vi "AB_Convert_To_Relative_Path.vi"(11 "absolute path":path) -> (3 "relative path":path)   [LabVIEW 2020]
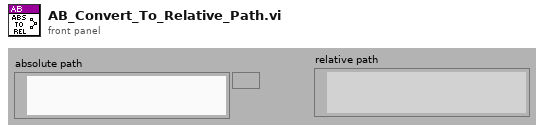
[diagram p1: front panel]
types:
  T1 = enum32{"invalid OS target", "Mac OS", "Windows 3.1", "Windows 95/NT", "Solaris 1", "Solaris 2", "HP-UX", "PowerMAX", "Linux", "Irix", "Rhapsody", "BeOS", "AIX", "OSF1", "VxWorks", "PharLap", "Carbon", "RTX", "Windows x64", "Linux x64", "Mac OS X x64"}
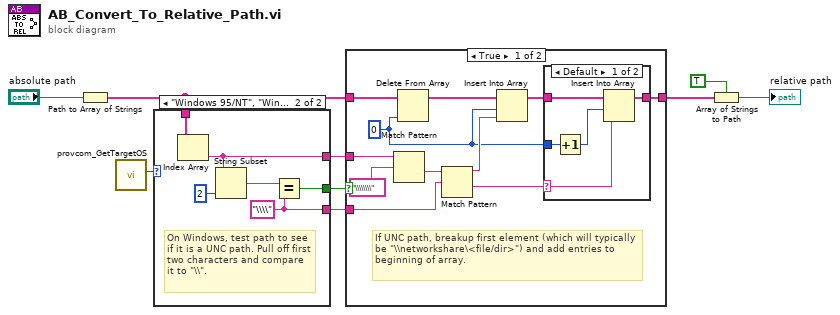
[diagram p0: block diagram]
diagram:
  n1 = Path to Array of Strings(0:"absolute path") -> (2:w7:string[])  [unwired: 1 out]
  n2 = call <resource>:"provcom_GetTargetOS.vi"() -> ("App.TargetOS"=w1:T1)  [unwired: 11 out]
  n3 = case shown="\"Windows 95/NT\", \"Windows x64\"" w1 {
    tunnel: [_ w13] -> w8
    tunnel: w7 -> [_ w12]
    tunnel: [_ w11] -> w5
    tunnel: [_ w10] -> w2
    frame Default {
    }
    frame "Windows 95/NT", "Windows x64" {
      w10 = "\\\\" ("regular expression")
      # "On Windows, test path to see if it is a UNC path. Pull off first two characters and compare it to \"\\\\\"."
      n4 = Index Array(array=w12) -> (element=w11:string)  [unwired: 1 in]
      n5 = String Subset(string=w11, length (rest)=2 ("length (rest)")) -> (substring=w14:string)  [unwired: 1 in]
      n6 = Equal?(x=w14, y=w10) -> (x = y?=w13:bool)
    }
  }
  n7 = case shown="True" w8 {
    tunnel: w7 -> [w26 w33]
    tunnel: [w17 w33] -> w6
    tunnel: w5 -> [w24 _]
    tunnel: w2 -> [w20 _]
    frame True {
      w16 = 0 ("index")
      # "If UNC path, breakup first element (which will typically be \"\\\\networkshare\\<file/dir>\") and add entries to beginning of array."
      n8 = Match Pattern(string=w24, regular expression="\\\\\\\\") -> (after substring=w23:string)  [unwired: 1 in, 3 out]
      n9 = Delete From Array(array=w26, index=w16) -> (array with subset deleted=w25:string[])  [unwired: 1 in, 1 out]
      n10 = Match Pattern(string=w23, regular expression=w20) -> (before substring=w22:string, after substring=w18:string)  [unwired: 1 in, 2 out]
      n11 = Insert Into Array(array=w25, index=w16, new element=w22) -> (w19:string[])
      n12 = case shown="Default" w18 {
        selector: w18 -> [w29 _]
        tunnel: w19 -> [w31 w32]
        tunnel: [w30 w32] -> w17
        tunnel: w16 -> [w28 _]
        frame Default {
          n13 = Increment(x=w28) -> (x+1=w27:i32)
          n14 = Insert Into Array(array=w31, index=w27, new element=w29) -> (w30:string[])
        }
        frame "" {
        }
      }
    }
    frame False {
    }
  }
  n15 = Array of Strings to Path(0:w6, 1:TRUE ("relative")) -> (2:→"relative path":path)
